vi "Configure.vi"(0 "SG Path Power Meter Accessor in":refnum<class "SG Path PM Accessor Base.lvclass">, 5 "frequency":dbl=50000000.0, 11 "error in (no error)":errorcluster) -> (4 "SG Path Power Meter Accessor out":refnum<class "SG Path PM Accessor Base.lvclass">, 15 "error out":errorcluster)   [LabVIEW 2023, in "RFFixtureCharact.Instruments.lvlib" / "SG Path PM Accessor Base.lvclass"]
uses:
  SG Path PM Accessor Base.lvclass
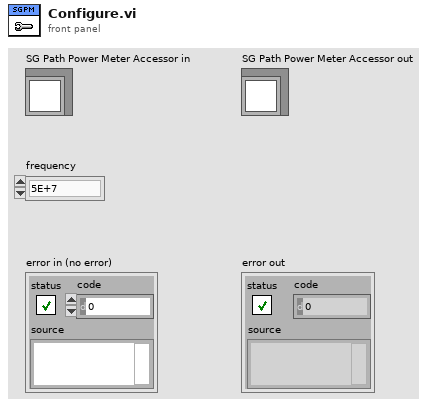
[diagram p1: front panel]
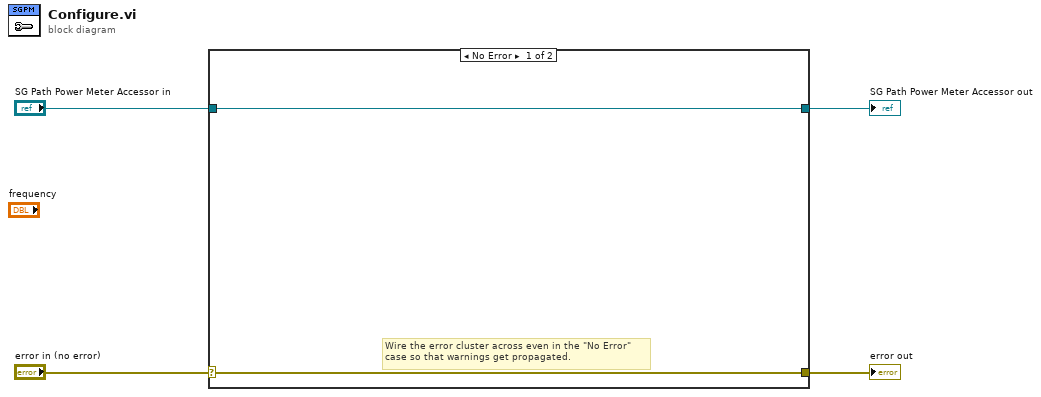
[diagram p0: block diagram]
diagram:
  n1 = case shown="No Error" "error in (no error)" {
    selector: "error in (no error)" -> [w5 w8]
    tunnel: [w5 w8] -> w3
    tunnel: [w6 w7] -> w1
    tunnel: "SG Path Power Meter Accessor in" -> [w6 w7]
    frame No Error {
      # "Wire the error cluster across even in the \"No Error\"\ncase so that warnings get propagated."
    }
    frame Error {
    }
  }
  "error out" <- w3
  "SG Path Power Meter Accessor out" <- w1
